vi "fpga_Phasor Measurement (P Class).vi"(0 "resampled data":T3, 1 "number of channels":T2=1 items=["1"=1, "2"=2, "3"=3, "4"=4, "5"=5, "6"=6, "7"=7, "8"=8, "9"=9, "10"=10, "11"=11, "12"=12, "13"=13, "14"=14, "15"=15, "16"=16], 5 "freq time difference [s]":fxp<+,18,-4>, 9 "input valid? (T)":bool=TRUE, 12 "ready for output? (T)":bool=TRUE) -> (4 "output data":T1 {"timestamp [s]" format="%#.6g"; "phase [pi]" format="%#.6g"}, 10 "output valid?":bool, 14 "ready for input?":bool)   [LabVIEW 2013, in "NI_EP_PMU_FPGA.lvlib"]
doc: "Computes the instantaneous magnitude, phase, and frequency values of the fundamental frequency component, at an output rate of 24 samples per cycle. You must use the FPGA Resampling VI to resample even-time-spaced voltage and current signals into even-angle-spaced signals before running this VI."
uses:
  <vilib>/addons/Electrical Power/PMU/NI_EP_PMU_FPGA.lvlib
  <vilib>/addons/Electrical Power/PQ/Resampling/FPGA/subVIs/fpga_Resampled.ctl
  <vilib>/addons/Electrical Power/PQ/Resampling/FPGA/subVIs/fpga_NofCH.ctl
  <vilib>/addons/Electrical Power/PMU/FPGA/subVIs/fpga_OutputDataType.ctl
  <vilib>/addons/Electrical Power/PQ/Resampling/NI_EP_Resample_FPGA.lvlib
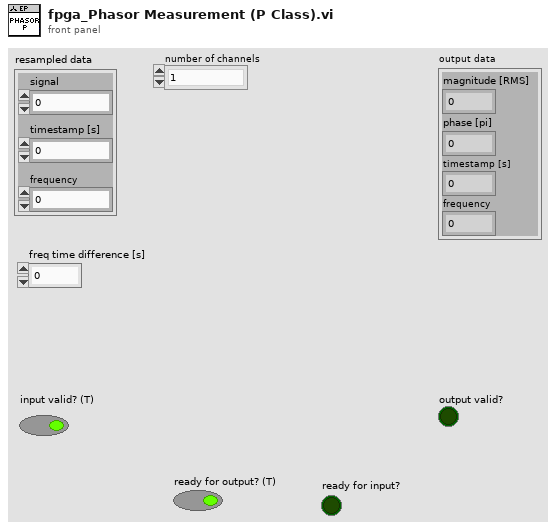
[diagram p1: front panel]
types:
  T1 = typedef "NI_EP_PMU_FPGA.lvlib/fpga_OutputDataType.ctl" = cluster{"magnitude [RMS]":fxp<+,32,6>, "phase [pi]":fxp<+/-,32,2>, "timestamp [s]":fxp<+,64,32>, "frequency":fxp<+,32,8>}
  T2 = typedef "NI_EP_Resample_FPGA.lvlib/fpga_NofCH.ctl" = u8
  T3 = typedef "NI_EP_Resample_FPGA.lvlib/fpga_Resampled.ctl" = cluster{"signal":fxp<+/-,32,3>, "timestamp [s]":fxp<+,64,32>, "frequency":fxp<+,32,8>}
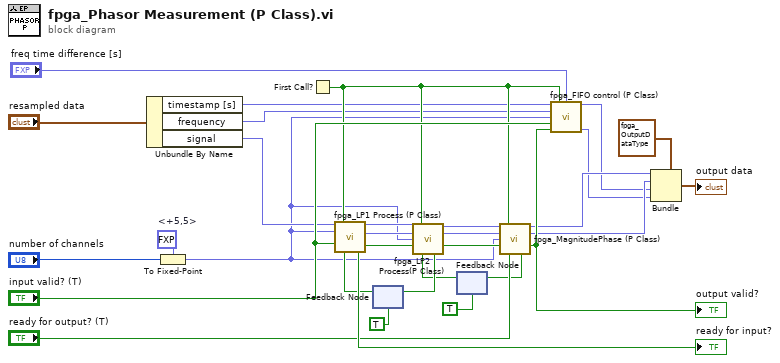
[diagram p0: block diagram]
diagram:
  w9 = fxp<+,5,5> 0.0  # <+5,5>
  n1 = Unbundle By Name("resampled data") -> ("timestamp [s]"=w12:fxp<+,64,32>, "frequency"=w10:fxp<+,32,8>, "signal"=w11:fxp<+/-,32,3>)
  n2 = To Fixed-Point(fixed-point type=w9, number="number of channels") -> (fixed-point=w8:fxp<+,5,5>)
  n3 = First Call?() -> (First Call?: T/F=w13:bool)
  n4 = feedback #1(TRUE ("ready for input")) -> (w22:bool)
  n5 = call <vilib>:"fpga_LP1 Process (P Class).vi"("input data"=w11, "reset"=w13, "Ch"=w8, "input valid"="input valid? (T)", "ready for output"=w22) -> ("re"=w25:fxp<+/-,32,5>, "im"=w24:fxp<+/-,32,5>, "output valid"=w21:bool, "ready for input"=→"ready for input?":bool)  [unwired: 7 in]
  n6 = feedback #2(TRUE ("ready for input")) -> (w15:bool)
  n7 = call <vilib>:"fpga_LP2 Process(P Class).vi"("re"=w25, "reset"=w13, "im"=w24, "#Ch"=w8, "input valid"=w21, "ready for output"=w15) -> ("re filtered"=w19:fxp<+/-,32,6>, "im filtered"=w18:fxp<+/-,32,6>, "output valid"=w17:bool, "ready for input"=w23:bool)  [unwired: 6 in]
  n8 = feedback-in #1(w23) -> ()
  n9 = call <vilib>:"fpga_MagnitudePhase (P Class).vi"("re"=w19, "reset"=w13, "im"=w18, "Ch"=w8, "input valid"=w17, "ready for output"="ready for output? (T)") -> ("rms magnitude"=w7:fxp<+,32,6>, "phase"=w6:fxp<+/-,32,2>, "output valid"=w28:bool, "ready for input"=w16:bool)  [unwired: 6 in]
  "output valid?" <- w28
  n10 = feedback-in #2(w16) -> ()
  n11 = call <vilib>:"fpga_FIFO control (P Class).vi"("Time stamp"=w12, "reset"=w13, "freq time difference [s]"="freq time difference [s]", "Frequency"=w10, "#ch"=w8, "PMU VI input valid"="input valid? (T)", "PMU VI output valid"=w28) -> ("Time Stamp out"=w5:fxp<+,64,32>, "Frequency output"=w4:fxp<+,32,8>)  [unwired: 7 in]
  n12 = Bundle(cluster=T1 {"magnitude [RMS]"=0.0, "phase [pi]"=0.0, "timestamp [s]"=0.0, "frequency"=0.0} ("output data"), "magnitude [RMS]"=w7, "phase [pi]"=w6, "timestamp [s]"=w5, "frequency"=w4) -> (→"output data":T1)
